vi "Channel Message Handler.vi"() -> ()   [LabVIEW 2019]
doc: "This template is for the Channel Message Handler design pattern.\n\nThe Event Handling Loop generates messages based on user interface actions.\n\nThe Message Handling Loop processes messages generated by the Event Handling Loop, or by other messages. The messages are string values, so new messages can be added easily to the Message Cases case structure in the Message Handling Loop. Each message cluster can also provide an optional value for Message Data, which is a variant that can be converted to whatever message-specific data is required."
uses:
  messages/MyMessage.lvclass/MyMessage.ctl
  <vilib>/ChannelSupport/Channel Message/Channel Message.lvclass/Channel Message.ctl
  <resource>/Channels/Messenger/Write With Abort.vi
  <extravilib>/ChannelInstances/Stream-str/Read With Abort.vi
  <resource>/Channels/Messenger/Read With Abort.vi
  <vilib>/ChannelSupport/Channel Message/Read ID.vi
  <extravilib>/ChannelInstances/Stream-str/Write With Abort.vi
  <extravilib>/ChannelInstances/Stream-str/EndpointRead.vi
  <extravilib>/ChannelInstances/Stream-str/Endpoint.vi
  messages/MyMessage.lvclass
  e:/builds/penguin/labview/branches/2019/dev/dist/vi.lib/ChannelSupport/Channel Message/Channel Message.lvclass
  <extravilib>/ChannelInstances/Stream-str/Instantiate.vi
  <extravilib>/ChannelInstances/Stream-str/)Channel.vi
  <resource>/ChannelSupport/_ChannelSupport/WaitIfNeeded.vi
  <resource>/Channels/Messenger/Instantiate.vi
  <resource>/Channels/Messenger/Endpoint.vi
  <resource>/Channels/Messenger/Messenger.lvlib
  <extravilib>/ChannelInstances/Stream-str.lvlib
panel:
  in  "Exit flag":bool
  out "Status":string
  in  "Do Something Else <Replace Me>":bool
  in  "Do Something <Replace Me>":bool
  in  "Exit":bool
  # "These controls have associated \"Value Changed\" events configured in the Event Structure on the diagram.\n\nReplace them (and reconfigure the Event Structure) with the controls you need for your application."
  # "This template is for the Channel Message Handler design pattern.\n\nSee the block diagram for more information on how to use this template."
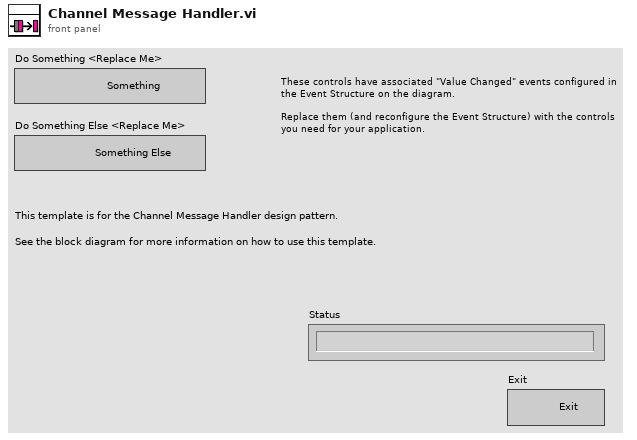
[diagram p1: front panel]
types:
  T1 = typedef "Messenger.lvlib/))Channel.ctl" = refnum<queue>
  T2 = typedef "Stream-str.lvlib/)Channel.ctl" = refnum<queue>
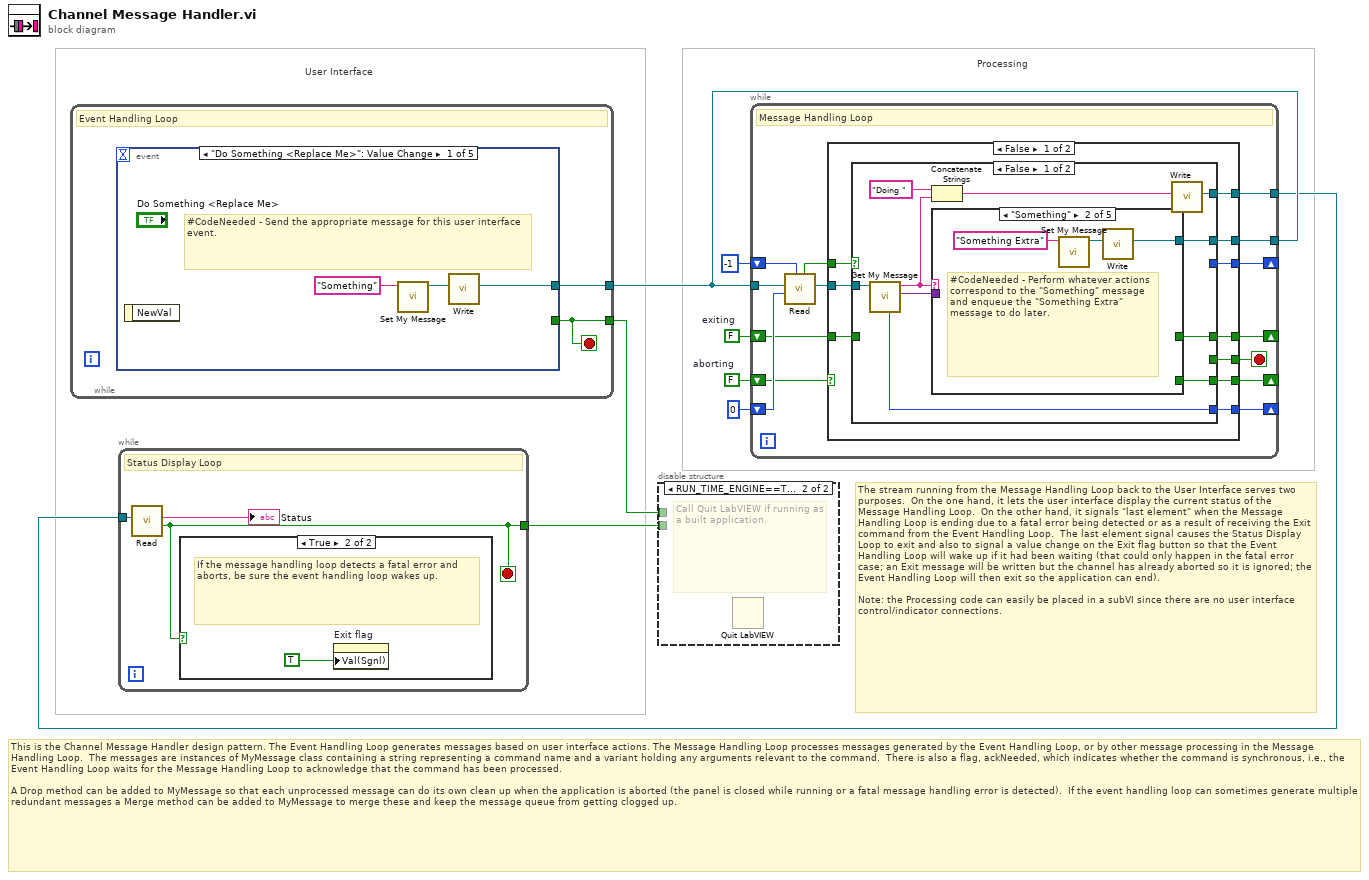
[diagram p0: block diagram]
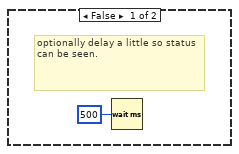
[diagram p2: hidden frame]
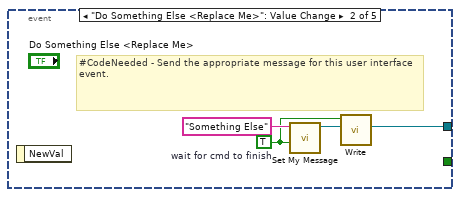
[diagram p4: hidden frame]
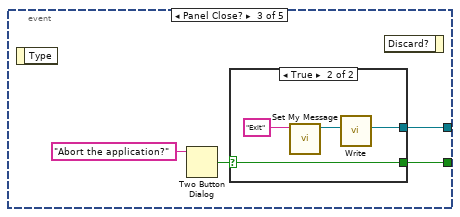
[diagram p5: hidden frame]
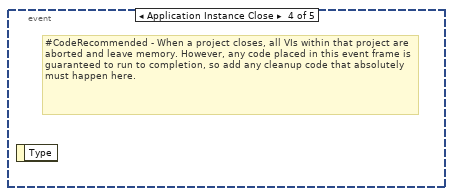
[diagram p7: hidden frame]
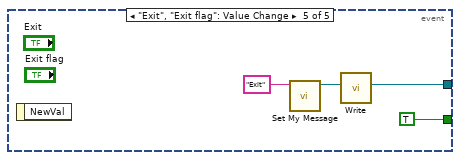
[diagram p8: hidden frame]
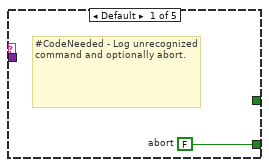
[diagram p9: hidden frame]
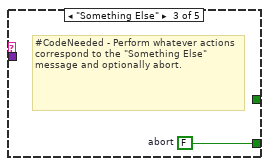
[diagram p10: hidden frame]
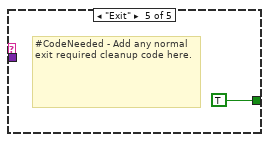
[diagram p12: hidden frame]
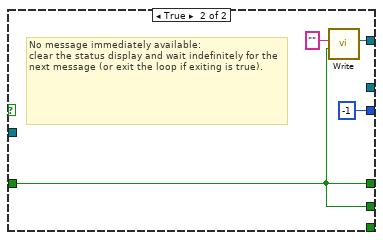
[diagram p13: hidden frame]
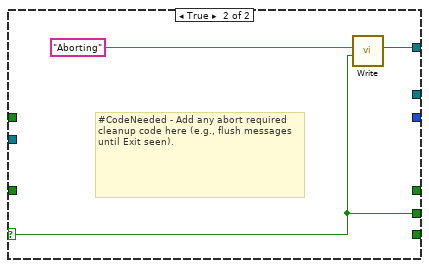
[diagram p14: hidden frame]
diagram:
  w1 = FALSE  # exiting
  w8 = FALSE  # aborting
  # "The stream running from the Message Handling Loop back to the User Interface serves two purposes.  On the one hand, it lets the user interface display the current status of the Message Handling Loop.  On the other hand, it signals \"last element\" when the Message Handling Loop is ending due to a fatal error being detected or as a result of receiving the Exit command from the Event Handling Loop.  The last element signal causes the Status Display Loop to exit and also to signal a value change on the Exit flag button so that the Event Handling Loop will wake up if it had been waiting (that could only happen in the fatal error case; an Exit message will be written but the channel has already aborted so it is ignored; the Event Handling Loop will then exit so the application can end).\n\nNote: the Processing code can easily be placed in a subVI since there are no user interface control/indicator connections."
  # "Processing"
  # "User Interface"
  # "This is the Channel Message Handler design pattern. The Event Handling Loop generates messages based on user interface actions. The Message Handling Loop processes messages generated by the Event Handling Loop, or by other message processing in the Message Handling Loop.  The messages are instances of MyMessage class containing a string representing a command name and a variant holding any arguments relevant to the command.  There is also a flag, ackNeeded, which indicates whether the command is synchronous, i.e., the Event Handling Loop waits for the Message Handling Loop to acknowledge that the command has been processed.\n\nA Drop method can be added to MyMessage so that each unprocessed message can do its own clean up when the application is aborted (the panel is closed while running or a fatal message handling error is detected).  If the event handling loop can sometimes generate multiple redundant messages a Merge method can be added to MyMessage to merge these and keep the message queue from getting clogged up."
  n1 = while {
    tunnel: [w10] -> w6
    tunnel: [w9] -> w4
    stop <- w9 stop-if-true
    # "Event Handling Loop"
    n2 = event shown="[0] \"Do Something <Replace Me>\": Value Change" {
      selector: _ -> [_ _ _ _ _]
      dyn-events: _ -> [_ _ _ _ _]
      timeout: _ -> [_ _ _ _ _]
      tunnel: [_ _ w18 _ TRUE] -> w9
      tunnel: [w11 w15 w20 _ w26] -> w10
      event "Do Something <Replace Me>": Value Change {
        # "#CodeNeeded - Send the appropriate message for this user interface event."
        n3 = event-data() -> ()  [unwired: 1 in, 1 out]
        n4 = call "Set My Message.vi"("command"="Something") -> ("MyMessage"=w12:refnum<class "MyMessage.lvclass">)  [unwired: 10 in]
        n5 = call <extravilib>:"Write.vi"("element"=w12) -> ("channel"=w11:T1)  [unwired: 8 in, 2 out]
      }
      event "Do Something Else <Replace Me>": Value Change {
        w14 = TRUE  # wait for cmd to finish
        # "#CodeNeeded - Send the appropriate message for this user interface event."
        n6 = event-data() -> ()  [unwired: 1 in, 1 out]
        n7 = call "Set My Message.vi"("ackNeeded"=w14, "command"="Something Else") -> ("MyMessage"=w16:refnum<class "MyMessage.lvclass">)  [unwired: 9 in]
        n8 = call <extravilib>:"Write.vi"("element"=w16, "wait for ack (F)"=w14) -> ("channel"=w15:T1)  [unwired: 7 in, 2 out]
      }
      event Panel Close? {
        n9 = event-data() -> ()  [unwired: 1 in, 1 out]
        n10 = Two Button Dialog(message="Abort the application?") -> (T button?=w19:bool)  [unwired: 2 in]
        n11 = case shown="True" w19 {
          selector: w19 -> [_ w24]
          tunnel: [_ w25] -> w20
          tunnel: [_ w24] -> w18
          frame False {
          }
          frame True {
            n12 = call "Set My Message.vi"("command"="Exit") -> ("MyMessage"=w22:refnum<class "MyMessage.lvclass">)  [unwired: 10 in]
            n13 = call <extravilib>:"Write.vi"("element"=w22) -> ("channel"=w25:T1)  [unwired: 8 in, 2 out]
          }
        }
        n14 = event-data() -> ()  [unwired: 2 in, 1 out]
      }
      event Application Instance Close {
        # "#CodeRecommended - When a project closes, all VIs within that project are aborted and leave memory. However, any code placed in this event frame is guaranteed to run to completion, so add any cleanup code that absolutely must happen here."
        n15 = event-data() -> ()  [unwired: 1 in, 1 out]
      }
      event "Exit", "Exit flag": Value Change {
        n16 = event-data() -> ()  [unwired: 1 in, 1 out]
        n17 = call "Set My Message.vi"("command"="Exit") -> ("MyMessage"=w27:refnum<class "MyMessage.lvclass">)  [unwired: 10 in]
        n18 = call <extravilib>:"Write.vi"("element"=w27) -> ("channel"=w26:T1)  [unwired: 8 in, 2 out]
      }
    }
  }
  n19 = while {
    tunnel: w6 -> [w43]
    shift-right: [w41] -> _
    shift-left: u32 0 ("id") -> [w40]
    shift-right: [w39] -> _
    shift-left: w8 -> [w30]
    tunnel: w6 -> [w38]
    tunnel: [w35] -> w5
    shift-right: [w33] -> _
    shift-left: -1 -> [w36]
    shift-right: [w32] -> _
    shift-left: w1 -> [w31]
    stop <- w37 stop-if-true
    # "Message Handling Loop"
    n20 = call <resource>:"Read.vi"("timeout in ms (-1)"=w36, "ack id (0)"=w40, "channel"=w43) -> ("element"=w42:refnum<class "Channel Message.lvclass">, "timed out?"=w34:bool)  [unwired: 6 in, 1 out]
    n21 = case shown="False" w30 {
      selector: w30 -> [_ w74]
      tunnel: w42 -> [w53 _]
      tunnel: [w52 _] -> w41
      tunnel: [w44 w74] -> w37
      tunnel: [w51 _] -> w39
      tunnel: [w50 _] -> w38
      tunnel: [w49 w76] -> w35
      tunnel: w34 -> [w48 _]
      tunnel: [w47 _] -> w33
      tunnel: [w46 _] -> w32
      tunnel: w31 -> [w45 _]
      frame False {
        n22 = case shown="False" w48 {
          tunnel: w53 -> [w63 _]
          tunnel: [w62 _] -> w52
          tunnel: [w60 _] -> w51
          tunnel: [w57 _] -> w50
          tunnel: [w55 w73] -> w49
          tunnel: [_ -1] -> w47
          tunnel: [w54 w70] -> w46
          tunnel: w45 -> [_ w70]
          tunnel: [_ w70] -> w44
          frame False {
            n23 = call "Get My Message.vi"("MyMessage"=w63) -> ("args"=w61:variant, "command"=w59:string, "id"=w62:u32)  [unwired: 7 in, 1 out]
            n24 = Concatenate Strings("Doing " ("string"), w59) -> (w56:string)
            n25 = case shown="\"Something\"" w59 {
              tunnel: w61 -> [_ _ _ _ _]
              tunnel: [_ _ _ _ TRUE] -> w54
              tunnel: [w64 _ w68 _ _] -> w60
              tunnel: [_ w65 _ _ _] -> w57
              frame Default {
                w64 = FALSE  # abort
                # "#CodeNeeded - Log unrecognized command and optionally abort."
              }
              frame "Something" {
                # "#CodeNeeded - Perform whatever actions correspond to the \"Something\" message and enqueue the \"Something Extra\" message to do later."
                n26 = call "Set My Message.vi"("command"="Something Extra") -> ("MyMessage"=w67:refnum<class "MyMessage.lvclass">)  [unwired: 10 in]
                n27 = call <extravilib>:"Write.vi"("element"=w67) -> ("channel"=w65:T1)  [unwired: 8 in, 2 out]
              }
              frame "Something Else" {
                w68 = FALSE  # abort
                # "#CodeNeeded - Perform whatever actions correspond to the \"Something Else\" message and optionally abort."
              }
              frame "Something Extra" {
                # "#CodeNeeded - Perform whatever actions correspond to the \"Something Extra\" message."
              }
              frame "Exit" {
                # "#CodeNeeded - Add any normal exit required cleanup code here."
              }
            }
            n28 = call <extravilib>:"Write.vi"("element"=w56) -> ("channel"=w55:T2)  [unwired: 8 in, 2 out]
          }
          frame True {
            # "No message immediately available:\nclear the status display and wait indefinitely for the next message (or exit the loop if exiting is true)."
            n29 = call <extravilib>:"Write.vi"("last element? (F)"=w70, "element"="") -> ("channel"=w73:T2)  [unwired: 7 in, 2 out]
          }
        }
      }
      frame True {
        # "#CodeNeeded - Add any abort required cleanup code here (e.g., flush messages until Exit seen)."
        n30 = call <extravilib>:"Write.vi"("last element? (F)"=w74, "element"="Aborting") -> ("channel"=w76:T2)  [unwired: 7 in, 2 out]
      }
    }
  }
  n31 = while {
    tunnel: w5 -> [w79]
    tunnel: [w77] -> w3
    stop <- w77 stop-if-true
    # "Status Display Loop"
    n32 = call <resource>:"Read.vi"("channel"=w79) -> ("last element?"=w77:bool, "element"=→"Status":string)  [unwired: 6 in, 3 out]
    n33 = case shown="True" w77 {
      frame False {
        # "optionally delay a little so status can be seen."
        n34 = Wait (ms)(milliseconds to wait=u32 500) -> ()  [unwired: 1 out]
      }
      frame True {
        # "If the message handling loop detects a fatal error and aborts, be sure the event handling loop wakes up."
        n35 = property on="Exit flag" class="Bool (strict)"("Val(Sgnl)"=TRUE) -> ()  [unwired: 2 in, 2 out]
      }
    }
  }
  n36 = disable-structure shown="RUN_TIME_ENGINE==True" {
    disable-tunnel: w4 -> [_ _]
    disable-tunnel: w3 -> [_ _]
    frame condition #0 (active) {
    }
    frame condition #1 {
      # "Call Quit LabVIEW if running as a built application."
      n37 = Quit LabVIEW() -> ()  [unwired: 1 in]
    }
  }
